vi "Read Daq Channels.vi"(6 "DisableDaqRead":bool, 8 "error_in":errorcluster, 10 "nSamples (100)":i32=100, 11 "task in":refnum<k21>) -> (0 "error out":errorcluster, 1 "Wfm data (NChanNSamp)":waveform(dbl)[](array[waveform]), 2 "DaqData":T1 {"Scans"."Data" format="%0.2f"; "AnalogVals" format="%.4f"}, 3 "task out":refnum<k21>, 5 "DAQ Latency?":bool)   [LabVIEW 2017]
doc: "Developed by: Kevin Thompson\nThompson Engineering\nthompson.engineering@comcast.net\n(510) 673-3614"
uses:
  TD AI Scalar DaqData--cluster.ctl
  <vilib>/DAQmx/read.llb/DAQmx Read (Analog 1D Wfm NChan NSamp).vi
  <vilib>/DAQmx/miscellaneous.llb/DAQmx Fill In Error Info.vi
  <userlib>/_OpenG.lib/error/error.llb/Filter Error Codes (Array)__ogtk.vi
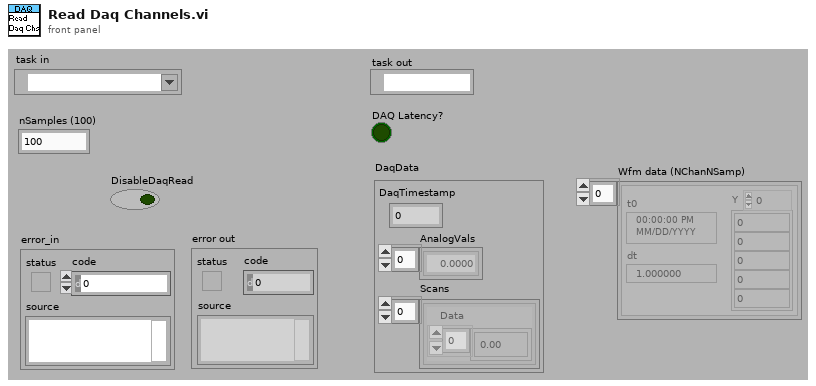
[diagram p1: front panel]
types:
  T1 = typedef "TD AI Scalar DaqData--cluster.ctl" = cluster{"DaqTimestamp":dbl, "AnalogVals":dbl[], "Scans":cluster{"Data":dbl[]}[]}
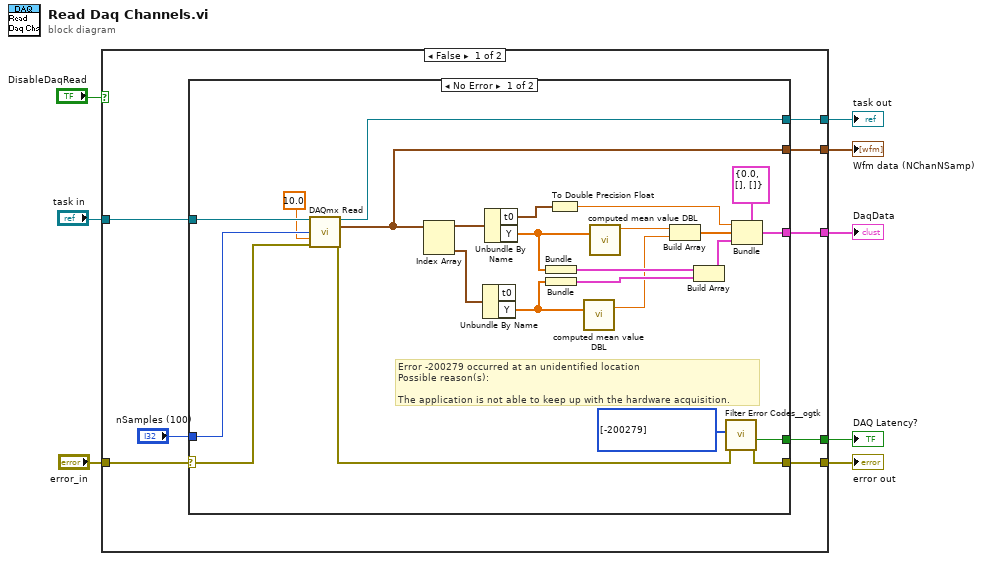
[diagram p0: block diagram]
diagram:
  n1 = case shown="False" "DisableDaqRead" {
    tunnel: "task in" -> [w16 w43]
    tunnel: [w15 _] -> w7
    tunnel: [w13 w43] -> w6
    tunnel: [w12 w44] -> w5
    tunnel: "error_in" -> [w11 w44]
    tunnel: [w10 _] -> w2
    tunnel: [w9 _] -> w1
    frame False {
      n2 = case shown="No Error" w11 {
        selector: w11 -> [w32 w41]
        tunnel: w16 -> [w37 w42]
        tunnel: [w27 w41] -> w12
        tunnel: [w33 _] -> w15
        tunnel: "nSamples (100)" -> [w36 _]
        tunnel: [w34 w42] -> w13
        tunnel: [w18 _] -> w10
        tunnel: [w17 _] -> w9
        frame No Error {
          # "Error -200279 occurred at an unidentified location\nPossible reason(s):\n\nThe application is not able to keep up with the hardware acquisition."
          n3 = call-poly <vilib>:"DAQmx Read.vi"("task/channels in"=w37, "number of samples per channel"=w36, "timeout"=10.0, "error in"=w32) -> ("task out"=w34:refnum<k21>, "data"=w17:waveform(dbl)[], "error out"=w31:errorcluster)  [unwired: 9 out]
          n4 = Index Array(array=w17) -> (element #1=w40:waveform(dbl), element #2=w29:waveform(dbl))  [unwired: 2 in]
          n5 = Unbundle By Name(w29) -> ("Y"=w25:dbl[])  [unwired: 1 out]
          n6 = Unbundle By Name(w40) -> ("t0"=w39:timestamp, "Y"=w26:dbl[])
          n7 = Bundle("Y"=w26) -> (w24:cluster{"Y":dbl[]})  [unwired: 1 in]
          n8 = Bundle("Y"=w25) -> (w23:cluster{"Y":dbl[]})  [unwired: 1 in]
          n9 = To Double Precision Float(number=w39) -> (double precision float=w38:dbl)
          n10 = call <vilib>:"computed mean value DBL.vi"("Array in"=w25) -> ("MeanValue"=w20:dbl)  [unwired: 1 out]
          n11 = call <vilib>:"computed mean value DBL.vi"("Array in"=w26) -> ("MeanValue"=w21:dbl)  [unwired: 1 out]
          n12 = Build Array(w21, w20) -> (w19:dbl[])
          n13 = Build Array(w24, w23) -> (w22:cluster{"Y":dbl[]}[])
          n14 = call-poly <userlib>:"Filter Error Codes__ogtk.vi"("Error In"=w31, "Error Codes to Filter"=i32[] [-200279]) -> ("Error Out"=w27:errorcluster, "Error Filtered?"=w18:bool)  [unwired: 7 in, 1 out]
          n15 = Bundle(cluster=T1 {"DaqTimestamp"=0.0, "AnalogVals"=[], "Scans"=[]} ("DaqData"), "DaqTimestamp"=w38, "AnalogVals"=w19, "Scans"=w22) -> (w33:T1)
        }
        frame Error {
        }
      }
    }
    frame True {
    }
  }
  "error out" <- w5
  "DaqData" <- w7
  "task out" <- w6
  "DAQ Latency?" <- w2
  "Wfm data (NChanNSamp)" <- w1
